vi "Channel (Range) Specifier.vi"(0 "Buffer":T1(ring)=enum."All", 5 "Card":i32, 7 "Channel":i32, 9 "Num Channels":i32, 11 "error in":errorcluster) -> (4 "Channel (Range)":string, 15 "error out":errorcluster)   [LabVIEW 2018]
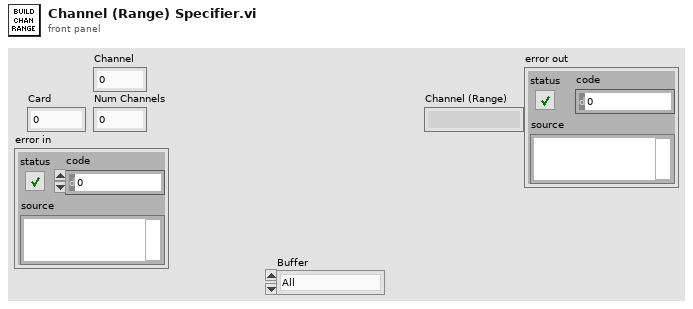
[diagram p1: front panel]
types:
  T1 = enum16{"Monitor", "Demand", "Backup", "All", "None"}
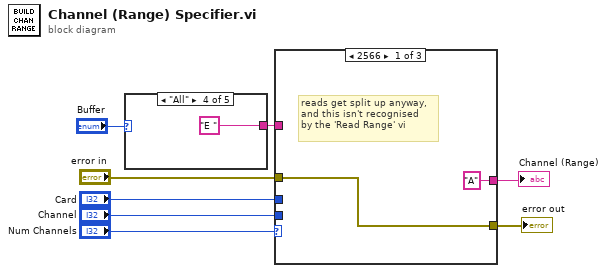
[diagram p0: block diagram]
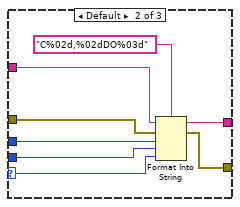
[diagram p2: hidden frame]
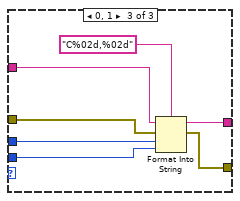
[diagram p3: hidden frame]
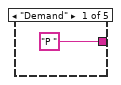
[diagram p4: hidden frame]
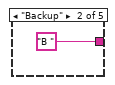
[diagram p5: hidden frame]
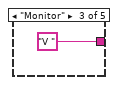
[diagram p6: hidden frame]
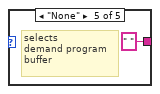
[diagram p7: hidden frame]
diagram:
  n1 = case shown="\"All\"" "Buffer" {
    tunnel: ["P " "B " "V " "E " " "] -> w4
    frame "Demand" {
    }
    frame "Backup" {
    }
    frame "Monitor" {
    }
    frame "All" {
    }
    frame "None" {
      # "selects \ndemand program\nbuffer"
    }
  }
  n2 = case shown="2566" "Num Channels" {
    selector: "Num Channels" -> [_ w16 _]
    tunnel: ["A" w22 w29] -> w8
    tunnel: [w14 w21 w28] -> w7
    tunnel: "error in" -> [w14 w20 w27]
    tunnel: w4 -> [_ w19 w26]
    tunnel: "Card" -> [_ w18 w25]
    tunnel: "Channel" -> [_ w17 w24]
    frame 2566 {
      # "reads get split up anyway,\nand this isn't recognised\nby the 'Read Range' vi"
    }
    frame Default {
      n3 = Format Into String(format string="C%02d,%02dDO%03d", initial string=w19, error in=w20, w18, w17, w16) -> (resulting string=w22:string, error out=w21:errorcluster)
    }
    frame 0, 1 {
      n4 = Format Into String(format string="C%02d,%02d", initial string=w26, error in=w27, w25, w24) -> (resulting string=w29:string, error out=w28:errorcluster)
    }
  }
  "Channel (Range)" <- w8
  "error out" <- w7
